vi "Extract Synchronous Data.vi"(8 "error in 2":errorcluster, 11 "Variant":variant) -> (0 "error in":errorcluster, 1 "Data Out":variant, 3 "notifier out":refnum<notifier>)   [LabVIEW 2021, in "Architecture.lvlib"]
doc: "This method extracts synchronous data from a message data to sepparate it into data and Callback ref. Use this Method to process data coming from a message in the destination module. \n\nUse the notifier to send a response to the sender module and unblock it."
uses:
  Architecture.lvlib
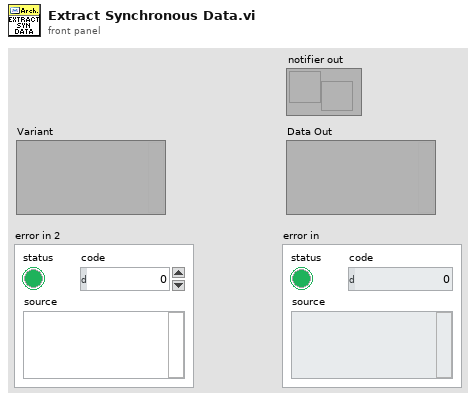
[diagram p1: front panel]
types:
  T1 = cluster{"Data":variant, "notifier out":refnum<notifier>}
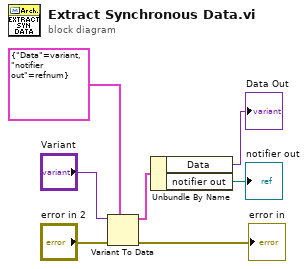
[diagram p0: block diagram]
diagram:
  n1 = Variant To Data(error in="error in 2", type=T1 {"Data"=variant, "notifier out"=refnum} ("output cluster"), Variant="Variant") -> (data=w5:T1, error out=→"error in":errorcluster)
  n2 = Unbundle By Name(w5) -> ("Data"=→"Data Out":variant, "notifier out"=→"notifier out":refnum<notifier>)
